vi "test_subvi.vi"(9 "Numeric 4":dbl, 10 "Numeric 3":dbl, 11 "Numeric in":dbl) -> (3 "Numeric out":dbl)   [LabVIEW 2019]
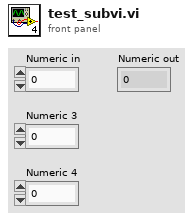
[diagram p1: front panel]
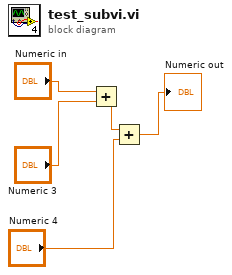
[diagram p0: block diagram]
diagram:
  n1 = Add(x="Numeric in", y="Numeric 3") -> (x+y=w3:dbl)
  n2 = Add(x=w3, y="Numeric 4") -> (x+y=→"Numeric out":dbl)
